vi "Technosoft_Standalone.vi"() -> ()   [LabVIEW 2011]
panel:
  out "return name":string="msr"
  out "connect OK":bool
  out "baud blank=9600, till=57600":i32=57600
  out "error out":errorcluster
  in  "stop":bool
  out "Binary":u16 format="%b"
  out "msr":bool[](array[boolean])
  out "return":dbl=nan
  in  "Run":bool[](array[boolean])=[FALSE, FALSE, FALSE, FALSE, FALSE, FALSE, FALSE, FALSE, FALSE, FALSE, FALSE, FALSE, FALSE, FALSE, FALSE, FALSE, FALSE, FALSE, FALSE, FALSE, FALSE, FALSE, FALSE]
  in  "commands":cluster{"command":string, "Value":dbl}[](array[cluster])=[{"command"="endinit", "Value"=0.0}, {"command"="axison", "Value"=0.0}, {"command"="cspd=", "Value"=-30.0}, {"command"="mode sp", "Value"=0.0}, {"command"="?mer", "Value"=0.0}, {"command"="?msr", "Value"=0.0}, {"command"="sap", "Value"=-1234.0}, {"command"="cpa", "Value"=0.0}, {"command"="mode pp3", "Value"=0.0}, {"command"="cpos=", "Value"=1923460.0}, {"command"="upd", "Value"=0.0}, {"command"="stop", "Value"=0.0}, {"command"="?tpos", "Value"=0.0}, {"command"="till_speed2=", "Value"=100.0}, {"command"="till_homespeed=", "Value"=100.0}, {"command"="goto tillcal", "Value"=0.0}, {"command"="goto tillrange", "Value"=0.0}, {"command"="till_speed=", "Value"=100.0}, {"command"="till_pos=", "Value"=123456.0}, {"command"="goto tillabs", "Value"=0.0}, {"command"="till_rel=", "Value"=123.0}, {"command"="goto tillrel", "Value"=0.0}, {"command"="?tille_runcurrent", "Value"=0.0}] {"Value" format="%#_8g"}
  in  "Axis #":u8=1
  in  "RS232-axis \n(blenk=255, TILL=1)\ncan be enterd after connect!":u8=1
  in  "Port, enter before start":refnum<visa-resource-name>="COM1"
  # "closes comport\notherwise use STOP"
  # "?mer bit6 is +limit, bit7 is -limit"
  # "6\n+lim"
  # "7\n-limit"
  # "9\nmotion\ncomplete"
  # "15\nUpdate"
  # "13\nAxisOn"
  # "0\ninit"
  # "--with TILL SW--\ntill_speed2=100\ntill_homespeed=50\ngoto tillcal\n?msr bit 7 is -switch\ntill_speed=800\n--move--\ntill_pos=12345\ngoto tillabs\n\ntill_rel=123\ngoto tillrel"
  # "1:x\n2:y\n3:obj?\n4:f1?\n5:f2?"
  # "---init new, empty board---\nendinit\naxison\ncspd=-50\nmode sp\nupd  <-move into switch: auxisoff\n?msr bit 9 or ?mer bit 7\nsap -1234\ncspd=200 (-50 can stay)\naxison (really needed?\ncpa\nmode pp3\n----move---\ncpos=12345\nupd"
  # "For debudding try also\nTechnosoftAskAll.vi!"
  # "1turn(400steps)=102400\n1 time=0,8ms\nspd=82=400step/s~1turn/s\n1A = 9027 (idmax,sbycrt)"
  # "?0x15002 read 5002 from EEPROM"
  # "Ignore warning 1073676294"
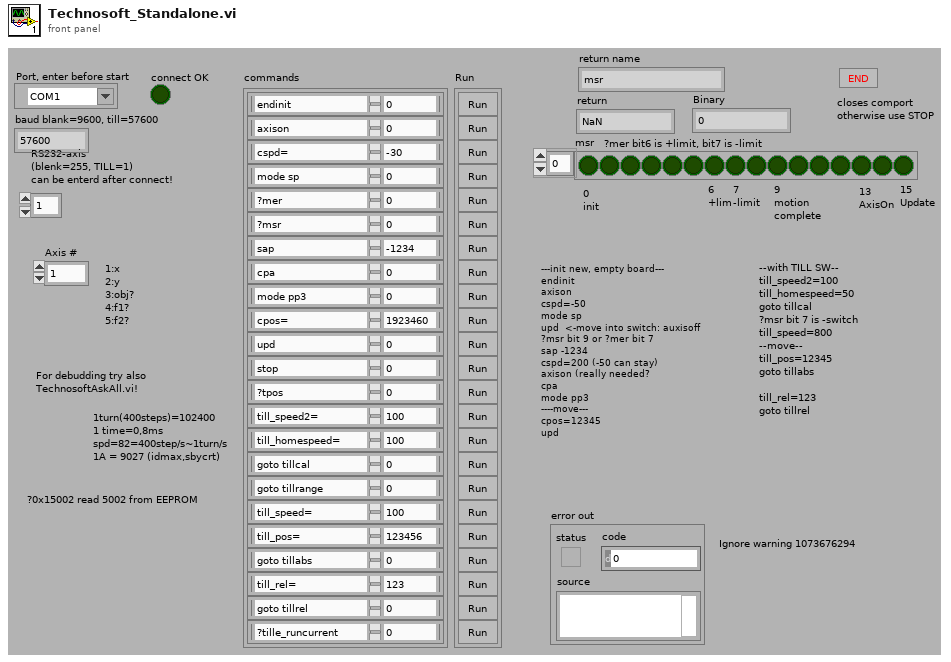
[diagram p1: front panel]
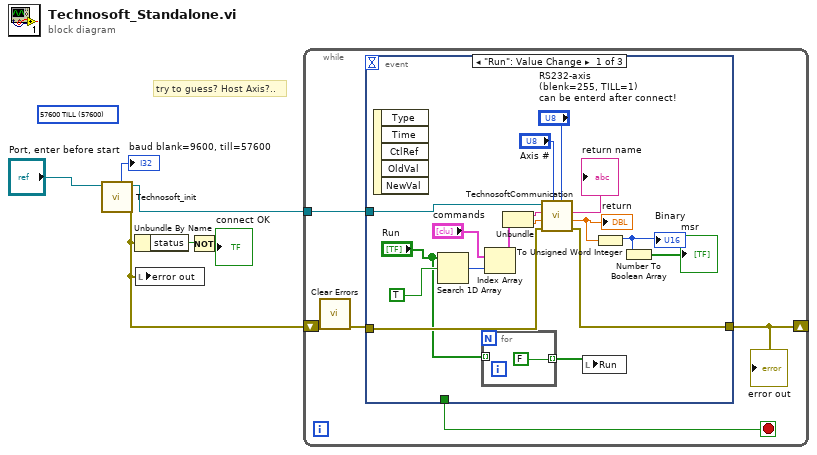
[diagram p0: block diagram]
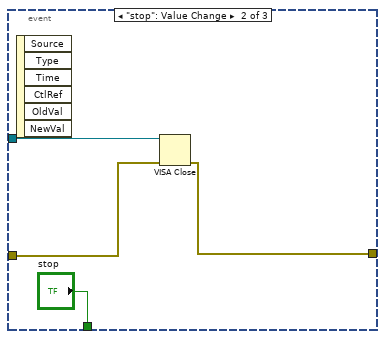
[diagram p2: hidden frame]
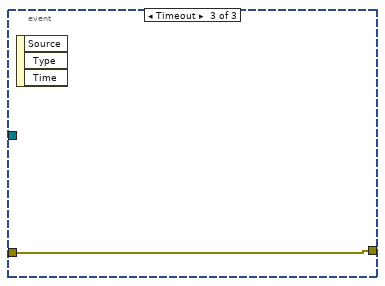
[diagram p3: hidden frame]
diagram:
  (unwired) u32 57600 items=[" 9600 new axis"=9600, "19200"=19200, "38400"=38400, "57600 TILL"=57600, "115200"=115200] ("baud")
  # "try to guess? Host Axis?.."
  n1 = call "Technosoft_init.vi"("VISA resource name"="Port, enter before start") -> ("error out"=w1:errorcluster, "VISA resource name out"=w5:refnum<visa-resource-name>, "Try baud"=→"baud blank=9600, till=57600":i32)  [unwired: 1 in, 7 out]
  n2 = Unbundle By Name(w1) -> ("status"=w3:bool)
  n3 = local write "error out"(w1) -> ()
  n4 = Not(x=w3) -> (.not. x?=→"connect OK":bool)
  n5 = while {
    shift-right: [w10] -> _
    shift-left: w1 -> [w9]
    tunnel: w5 -> [w8]
    stop <- w11 stop-if-true
    n6 = call <vilib>:"Clear Errors.vi"("error in (no error)"=w9) -> ("error out"=w7:errorcluster)  [unwired: 6 out]
    n7 = event shown="[0] \"Run\": Value Change" {
      selector: _ -> [_ _ _]
      dyn-events: _ -> [_ _ _]
      timeout: _ -> [_ _ _]
      tunnel: [_ "stop" _] -> w11
      tunnel: [w17 w31 w34] -> w10
      tunnel: w7 -> [w16 w32 w34]
      tunnel: w8 -> [w15 w30 _]
      event "Run": Value Change {
        n8 = event-data() -> ()  [unwired: 6 out]
        n9 = Search 1D Array(1D array="Run", element=TRUE) -> (index of element=w22:i32)  [unwired: 1 out]
        n10 = for {
          tunnel: "Run" -> [_] mode=indexing
          tunnel: [FALSE ("element")] -> w13 mode=indexing
        }
        n11 = Index Array(array="commands", index=w22) -> (element=w20:cluster{"command":string, "Value":dbl})
        n12 = Unbundle(w20) -> ("command"=w19:string, "Value"=w18:dbl)
        n13 = call "TechnosoftCommunication.vi"("RS232-axis"="RS232-axis \n(blenk=255, TILL=1)\ncan be enterd after connect!", "axis"="Axis #", "error in (no error)"=w16, "value"=w18, "command"=w19, "VISA resource name"=w15) -> ("error out"=w17:errorcluster, "return"=w25:dbl, "return name"=→"return name":string)  [unwired: 3 out]
        "return" <- w25
        n14 = local write "Run"(w13) -> ()
        n15 = To Unsigned Word Integer(number=w25) -> (unsigned 16bit integer=w26:u16)
        "Binary" <- w26
        n16 = Number To Boolean Array(number=w26) -> (Boolean array=→"msr":bool[])
      }
      event "stop": Value Change {
        n17 = event-data() -> ()  [unwired: 7 out]
        n18 = VISA Close(VISA resource name=w30, error in (no error)=w32) -> (error out=w31:errorcluster)
      }
      event Timeout {
        n19 = event-data() -> ()  [unwired: 4 out]
      }
    }
    "error out" <- w10
  }
